vi "iRobot Example - Remote Control.vi"() -> ()   [LabVIEW 2014]
doc: "Simplest example for streaming iRobot sensors."
uses:
  Advanced/UART/iRobot UART Port Type.ctl
  Sensor/Sensor Group 6.ctl
  Sensor/Bumps + Wheel Drops.ctl
  Sensor/Buttons.ctl
  Sensor/Charging State.ctl
  Sensor/Charging Sources Available.ctl
  Sensor/OI Mode.ctl
  Sensor/Cargo Bay Digital Inputs.ctl
  Sensor/Low-Side Driver + Wheel Overcurrent.ctl
panel:
  in  "UART port in":T1="ASRL1::INSTR"
  in  "stop":bool
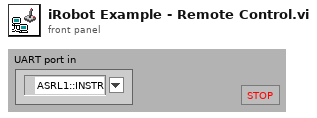
[diagram p1: front panel]
types:
  T1 = typedef "iRobot UART Port Type.ctl" = refnum<visa-resource-name>
  T2 = typedef "Sensor Group 6.ctl" = cluster{"Bumps + Wheel Drops":T3, "Wall":bool, "Cliff Left":bool, "Cliff Front Left":bool, "Cliff Front Right":bool, "Cliff Right":bool, "Wall Signal":u16, "Cliff Left Signal":u16, "Cliff Front Left Signal":u16, "Cliff Front Right Signal":u16, "Cliff Right Signal":u16, "Buttons":T4, "Virtual Wall":bool, "# Stream Packets":u8, "Requested Velocity (mm/s)":i16, "Requested Radius (mm)":i16, "Requested Right Wheel Velocity (mm/s)":i16, "Requested Left Wheel Velocity (mm/s)":i16, "Distance (mm)":i32, "Angle (deg)":i32, "Song Playing":bool, "Song Number":u8, "Charging State":T5, "Voltage (mV)":u16, "Current (mA)":i16, "Battery Temperature (deg C)":i8, "Battery Charge (mAh)":u16, "Battery Capacity (mAh)":u16, "Charging Sources":T6, "OI Mode":T7, "Digital Inputs":T8, "Drivers & Wheel Overcurrent":T9, "Analog Signal":u16, "Infrared":u8}
  T3 = typedef "Bumps + Wheel Drops.ctl" = cluster{"Wheeldrop Caster":bool, "Wheeldrop Left":bool, "Wheeldrop Right":bool, "Bump Left":bool, "Bump Right":bool}
  T4 = typedef "Buttons.ctl" = cluster{"Advance":bool, "Play":bool}
  T5 = typedef "Charging State.ctl" = enum16{"Not Charging", "Reconditioning Charging", "Full Charging", "Trickle Charging", "Waiting", "Charging Fault Condition"}
  T6 = typedef "Charging Sources Available.ctl" = cluster{"Internal Charger":bool, "Home Base":bool}
  T7 = typedef "OI Mode.ctl" = enum16{"Off", "Passive", "Safe", "Full"}
  T8 = typedef "Cargo Bay Digital Inputs.ctl" = cluster{"Digital Input 0":bool, "Digital Input 1":bool, "Digital Input 2":bool, "Digital Input 3":bool, "Device Detect":bool}
  T9 = typedef "Low-Side Driver + Wheel Overcurrent.ctl" = cluster{"Low-Side Driver 0":bool, "Low-Side Driver 1":bool, "Low-Side Driver 2":bool, "Left Wheel":bool, "Right Wheel":bool}
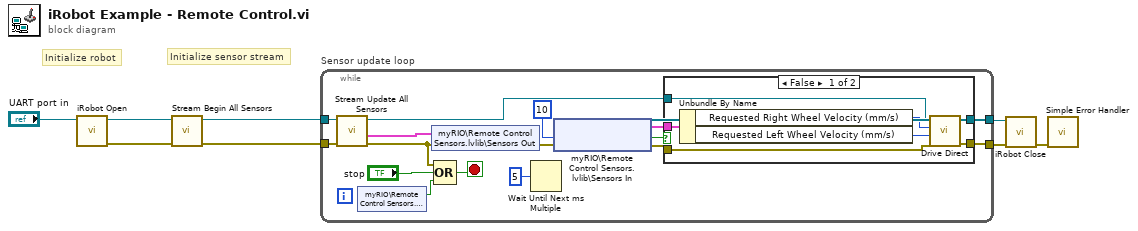
[diagram p0: block diagram]
diagram:
  # "Initialize sensor stream"
  # "Initialize robot"
  n1 = call "iRobot Open.vi"("UART port in"="UART port in") -> ("error out"=w6:errorcluster, "UART port out"=w8:T1)  [unwired: 9 in]
  n2 = call "Stream Begin All Sensors.vi"("error in"=w6, "UART port in"=w8) -> ("error out"=w5:errorcluster, "UART port out"=w7:T1)  [unwired: 8 in]
  n3 = while "Sensor update loop" {
    tunnel: w7 -> [w24]
    tunnel: [w12] -> w3
    tunnel: w5 -> [w23]
    tunnel: [w11] -> w4
    stop <- w21 stop-if-true
    n4 = call "Stream Update All Sensors.vi"("error in"=w23, "UART port in"=w24) -> ("error out"=w18:errorcluster, "sensors"=w17:T2, "UART port out"=w13:T1)  [unwired: 5 in, 2 out]
    n5 = shared-variable "myRIO\\Remote Control Sensors.lvlib\\Stop"() -> (w9:bool)  [unwired: 1 in, 1 out]
    n6 = shared-variable "myRIO\\Remote Control Sensors.lvlib\\Sensors Out"(w17, error in=w18) -> (error out=w19:errorcluster)
    n7 = Compound Arithmetic op=OR(w18, "stop", w9) -> (w21:bool)
    n8 = Wait Until Next ms Multiple(millisecond multiple=u32 5) -> ()  [unwired: 1 out]
    n9 = shared-variable "myRIO\\Remote Control Sensors.lvlib\\Sensors In"(error in=w19, 10 ("ms timeout (0)")) -> (w15:T2, error out=w10:errorcluster, w14:bool)
    n10 = case shown="False" w14 {
      tunnel: w15 -> [w29 _]
      tunnel: w13 -> [w28 w33]
      tunnel: [w27 w33] -> w12
      tunnel: [w26 w32] -> w11
      tunnel: w10 -> [w25 w32]
      frame False {
        n11 = Unbundle By Name(w29) -> ("Requested Right Wheel Velocity (mm/s)"=w30:i16, "Requested Left Wheel Velocity (mm/s)"=w31:i16)
        n12 = call "Drive Direct.vi"("error in"=w25, "Left Wheel Velocity (mm/s)"=w31, "Right Wheel Velocity (mm/s)"=w30, "UART port in"=w28) -> ("error out"=w26:errorcluster, "UART port out"=w27:T1)  [unwired: 6 in]
      }
      frame True {
      }
    }
  }
  n13 = call "iRobot Close.vi"("error in"=w4, "UART port in"=w3) -> ("error out"=w2:errorcluster)  [unwired: 9 in]
  n14 = call <vilib>:"Simple Error Handler.vi"("error in (no error)"=w2) -> ()  [unwired: 4 in, 5 out]
